vi "AMIMonitor.vi"() -> ()   [LabVIEW 2018]
uses:
  Global/Global Variables/Data_Display_global.vi
  Instrument_Setup.vi
panel:
  out "Numeric":i32
  out "Field set":bool
  out "Field rates set":bool=TRUE
  out "error out":errorcluster
  in  "error in (no error)":errorcluster
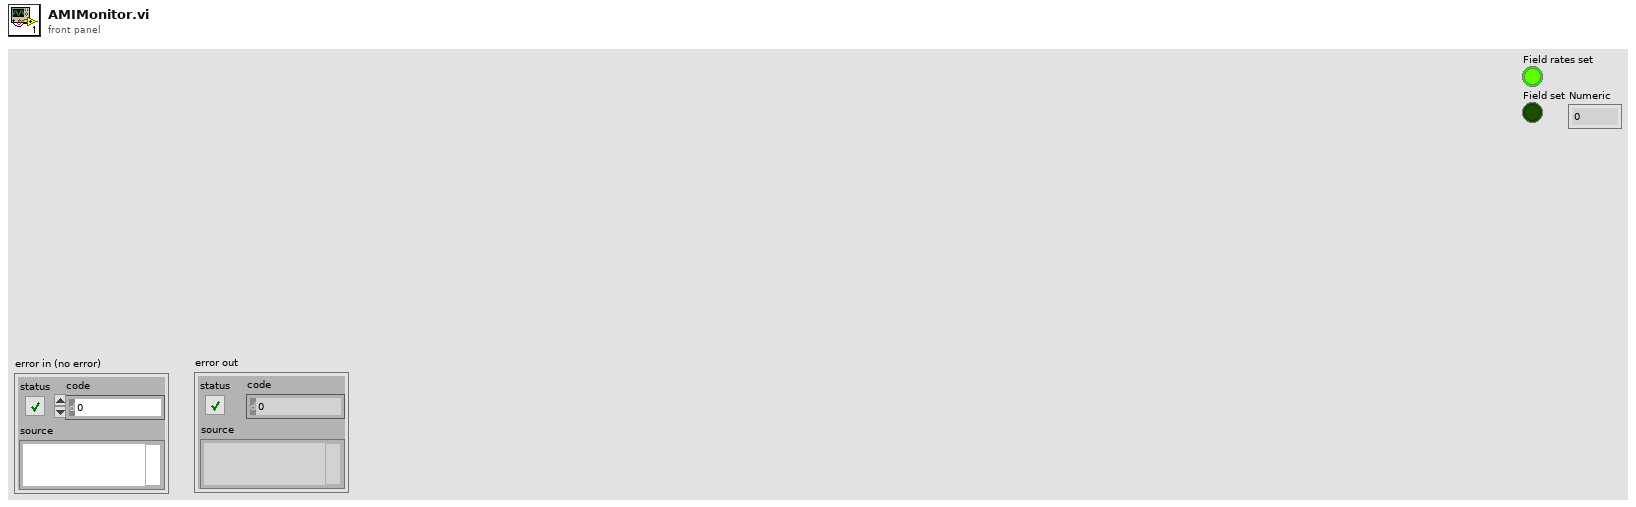
[diagram p1: front panel]
types:
  T1 = cluster{"GPIB address":i16, "GPIB bus":i16, "connection ID":refnum<k5>, "IP":string, "Active Comm Interface":u16, "Serial Port":refnum<visa-resource-name>, "Programmer Type":u16}
  T2 = cluster{"error":bool, "code":i32, "source":string}
  T3 = enum16{"", "RAMPING", "HOLDING", "PAUSED", "MANUAL UP", "MANUAL DOWN", "ZEROING CURRENT", "QUENCH DETECTED", "HEATING SWITCH", "AT ZER0", "COOLING SWITCH"}
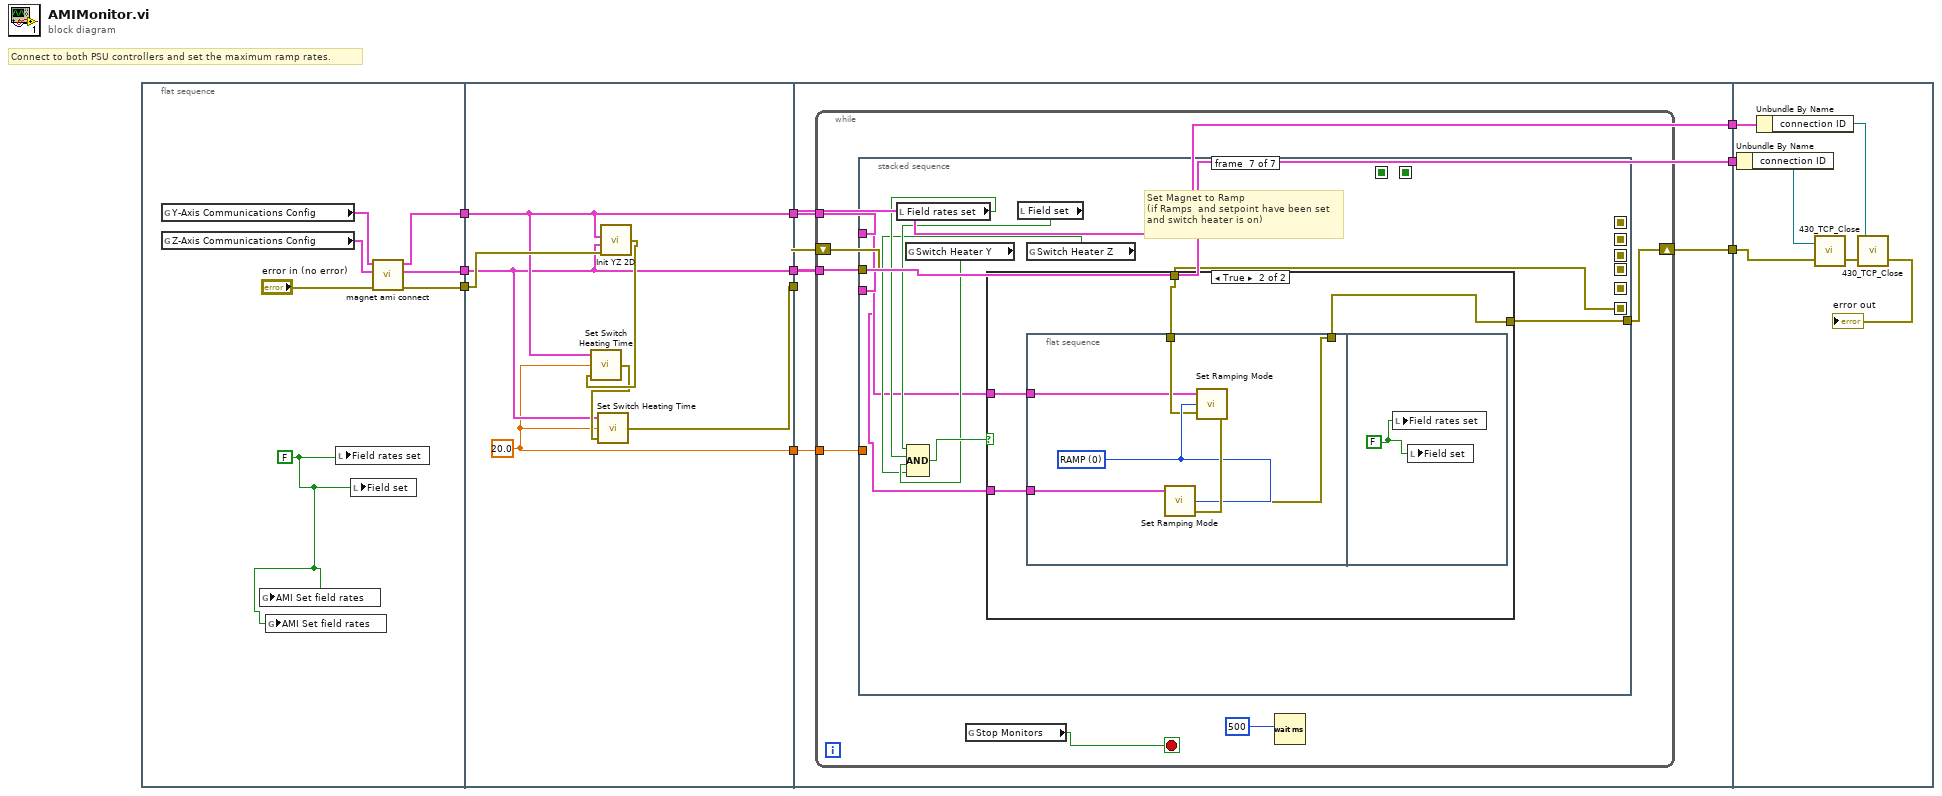
[diagram p0: block diagram]
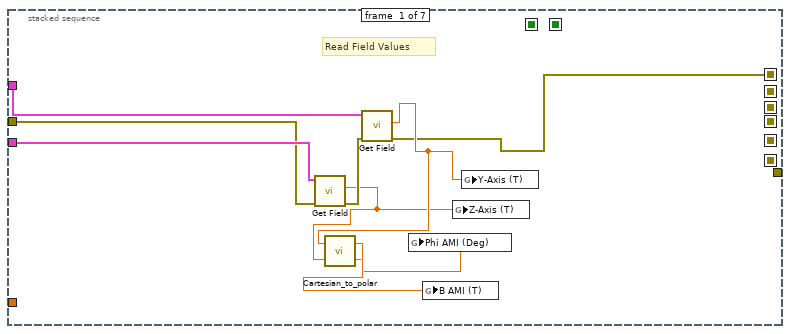
[diagram p2: hidden frame]
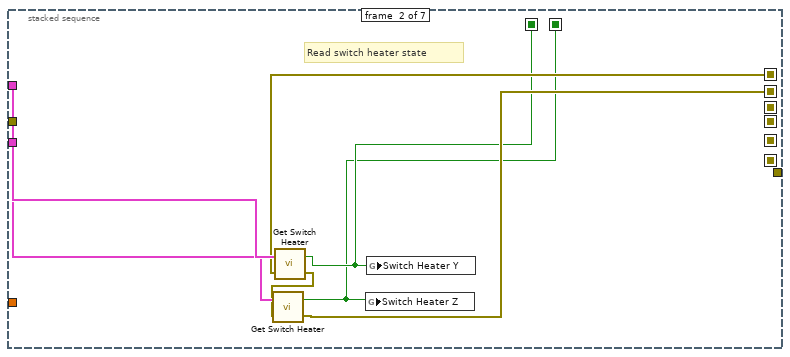
[diagram p3: hidden frame]
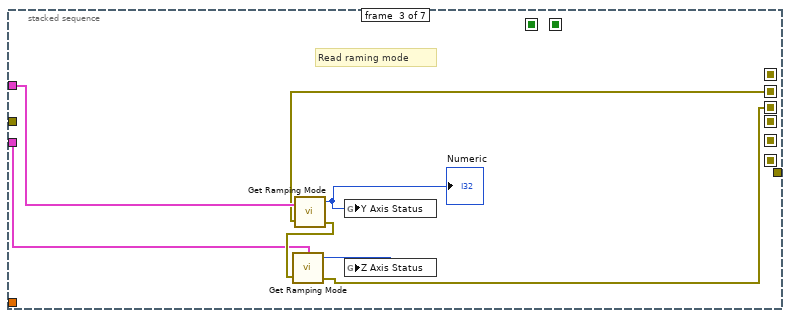
[diagram p4: hidden frame]
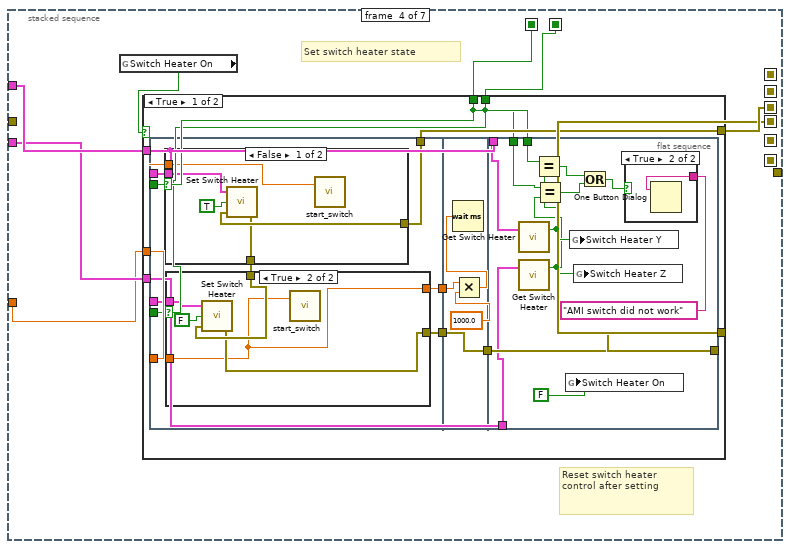
[diagram p5: hidden frame]
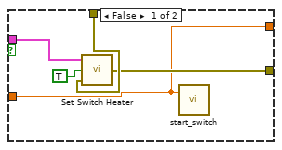
[diagram p6: hidden frame]
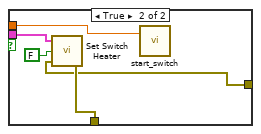
[diagram p7: hidden frame]
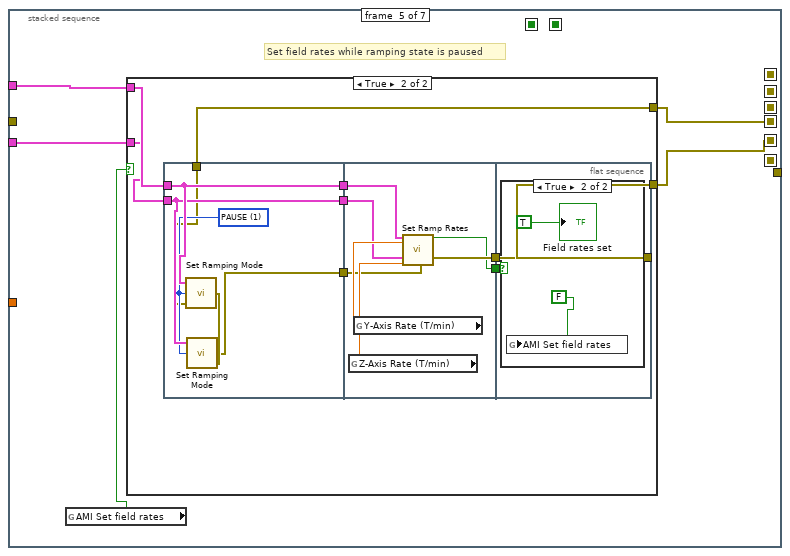
[diagram p10: hidden frame]
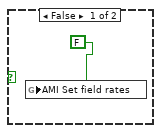
[diagram p12: hidden frame]
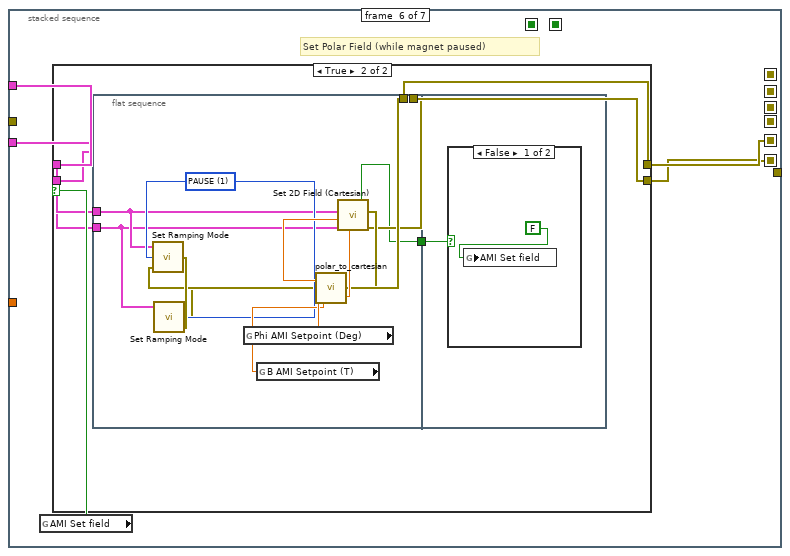
[diagram p13: hidden frame]
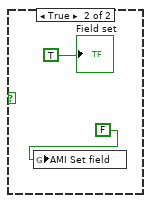
[diagram p15: hidden frame]
diagram:
  # "Connect to both PSU controllers and set the maximum ramp rates."
  n1 = flat-sequence {
    tunnel: [w14] -> w10
    tunnel: [w13] -> w8
    tunnel: [w12] -> w6
    tunnel: w10 -> [w23]
    tunnel: [w23] -> w9
    tunnel: w8 -> [w19]
    tunnel: [w19] -> w7
    tunnel: w6 -> [w24]
    tunnel: [w20] -> w5
    tunnel: [w18] -> w1
    tunnel: w9 -> [w28]
    tunnel: w7 -> [w27]
    tunnel: w5 -> [w29]
    tunnel: [w28] -> w4
    tunnel: [w27] -> w3
    tunnel: [w26] -> w2
    tunnel: w1 -> [w25]
    tunnel: w4 -> [w208]
    tunnel: w3 -> [w207]
    tunnel: w2 -> [w206]
    frame #0 {
      w11 = FALSE
      n2 = global read "Instrument_Setup.vi" "Y-Axis Communications Config"() -> (w17:T1)
      n3 = global read "Instrument_Setup.vi" "Z-Axis Communications Config"() -> (w16:T1)
      n4 = global write "Data_Display_global.vi" "AMI Set field rates"(w11) -> ()
      n5 = global write "Data_Display_global.vi" "AMI Set field rates"(w11) -> ()
      n6 = local write "Field rates set"(w11) -> ()
      n7 = local write "Field set"(w11) -> ()
      n8 = call "magnet ami connect.vi"("error in (no error)"="error in (no error)", "Z-Axis Communications Config"=w16, "Y-Axis Communications Config"=w17) -> ("error out"=w12:errorcluster, "Z-Axis Communications Config Out"=w13:T1, "Y-Axis Communications Config Out"=w14:T1)  [unwired: 6 in]
    }
    frame #1 {
      w18 = 20.0
      n9 = call "Init YZ 2D.vi"("error in"=w24, "Z-Axis Communications Config"=w19, "Y-Axis Communications Config"=w23) -> ("error out"=w22:T2)  [unwired: 7 in]
      n10 = call "Set Switch Heating Time.vi"("error in"=w22, "Switch Heating Time (sec)"=w18, "Communications Config"=w23) -> ("error out"=w21:T2)
      n11 = call "Set Switch Heating Time.vi"("error in"=w21, "Switch Heating Time (sec)"=w18, "Communications Config"=w19) -> ("error out"=w20:T2)
    }
    frame #2 {
      n12 = while {
        tunnel: w28 -> [w36]
        tunnel: w27 -> [w35]
        shift-right: [w30] -> w26
        shift-left: w29 -> [w34]
        tunnel: w25 -> [w31]
        stop <- w33 stop-if-true
        n13 = stacked-sequence {
          seq-local: [w37 _ _ _ _ _ _] -> [_ w50 _ _ _ _ _]
          seq-local: [_ _ _ w60 _ _ _] -> [_ _ _ _ w126 _ _]
          seq-local: [_ w48 _ _ _ _ _] -> [_ _ w55 _ _ _ _]
          seq-local: [_ w47 _ _ _ _ _] -> [_ _ _ w63 _ _ _]
          seq-local: [_ w46 _ _ _ _ _] -> [_ _ _ w62 _ _ _]
          seq-local: [_ _ w54 _ _ _ _] -> [_ _ _ w61 _ _ _]
          seq-local: [_ _ _ _ w125 _ _] -> [_ _ _ _ _ w159 _]
          seq-local: [_ _ _ _ _ w158 _] -> [_ _ _ _ _ _ w193]
          tunnel: w36 -> [w45 w52 w58 w66 w128 w162 w186]
          tunnel: w35 -> [w44 w51 w57 w65 w129 w161 w185]
          tunnel: w34 -> [w42 _ _ _ _ _ _]
          tunnel: w31 -> [_ _ _ w64 _ _ _]
          tunnel: [_ _ _ _ _ _ w192] -> w30
          frame #0 {
            # "Read Field Values"
            n14 = call "Get Field.vi"("Z-Axis Communications Config"=w44, "error in"=w42) -> ("Field(T)"=w40:dbl, "error out"=w43:T2)  [unwired: 4 in, 1 out]
            n15 = call "Get Field.vi"("Z-Axis Communications Config"=w45, "error in"=w43) -> ("Field(T)"=w41:dbl, "error out"=w37:T2)  [unwired: 4 in, 1 out]
            n16 = call "Cartesian_to_polar.vi"("Z-Axis (T)"=w40, "Y-Axis (T)"=w41) -> ("phi (deg)"=w38:dbl, "Radial (r) Field (T)"=w39:dbl)
            n17 = global write "Data_Display_global.vi" "Phi AMI (Deg)"(w38) -> ()
            n18 = global write "Data_Display_global.vi" "B AMI (T)"(w39) -> ()
            n19 = global write "Data_Display_global.vi" "Z-Axis (T)"(w40) -> ()
            n20 = global write "Data_Display_global.vi" "Y-Axis (T)"(w41) -> ()
          }
          frame #1 {
            # "Read switch heater state"
            n21 = call "Get Switch Heater.vi"("error in"=w50, "Communications Config"=w52) -> ("error out"=w49:T2, "Switch Heater Indicator"=w47:bool)
            n22 = call "Get Switch Heater.vi"("error in"=w49, "Communications Config"=w51) -> ("error out"=w48:T2, "Switch Heater Indicator"=w46:bool)
            n23 = global write "Data_Display_global.vi" "Switch Heater Z"(w46) -> ()
            n24 = global write "Data_Display_global.vi" "Switch Heater Y"(w47) -> ()
          }
          frame #2 {
            # "Read raming mode"
            n25 = call "Get Ramping Mode.vi"("Communications Config"=w58, "error in"=w55) -> ("Ramping Mode"=w53:T3, "error out"=w59:T2)  [unwired: 1 out]
            "Numeric" <- w53
            n26 = call "Get Ramping Mode.vi"("Communications Config"=w57, "error in"=w59) -> ("Ramping Mode"=w56:T3, "error out"=w54:T2)  [unwired: 1 out]
            n27 = global write "Data_Display_global.vi" "Y Axis Status"(w53) -> ()
            n28 = global write "Data_Display_global.vi" "Z Axis Status"(w56) -> ()
          }
          frame #3 {
            # "Reset switch heater \ncontrol after setting"
            # "Set switch heater state"
            n29 = global read "Data_Display_global.vi" "Switch Heater On"() -> (w67:bool)
            n30 = case shown="True" w67 {
              tunnel: w66 -> [w71 _]
              tunnel: w65 -> [w70 _]
              tunnel: w64 -> [w77 _]
              tunnel: w61 -> [w75 w124]
              tunnel: w63 -> [w69 _]
              tunnel: w62 -> [w68 _]
              tunnel: [w74 w124] -> w60
              frame True {
                n31 = flat-sequence {
                  tunnel: w71 -> [w86]
                  tunnel: w70 -> [w85]
                  tunnel: w77 -> [w82]
                  tunnel: [w83] -> w76
                  tunnel: w75 -> [w81]
                  tunnel: w69 -> [w80]
                  tunnel: w68 -> [w79]
                  tunnel: [w78] -> w73
                  tunnel: w76 -> [w110]
                  tunnel: w73 -> [w108]
                  tunnel: [w110] -> w72
                  tunnel: [w122] -> w74
                  tunnel: w72 -> [w122]
                  tunnel: w71 -> [w120]
                  tunnel: w70 -> [w119]
                  tunnel: w69 -> [w118]
                  tunnel: w68 -> [w117]
                  frame #0 {
                    n32 = case shown="False" w80 {
                      tunnel: w86 -> [w101 w105]
                      tunnel: w81 -> [w99 w102]
                      tunnel: [w98 w103] -> w84
                      tunnel: w82 -> [w97 w104]
                      frame False {
                        n33 = call "Set Switch Heater.vi"("error in"=w99, "Switch Heater Control"=TRUE, "Communications Config"=w101) -> ("error out"=w98:T2)
                        n34 = call "start_switch.vi"("Switch heater time"=w97) -> ()  [unwired: 2 in]
                      }
                      frame True {
                        n35 = call "Set Switch Heater.vi"("error in"=w102, "Switch Heater Control"=FALSE, "Communications Config"=w105) -> ("error out"=w103:T2)
                        n36 = call "start_switch.vi"("Switch heater time"=w104) -> ()  [unwired: 2 in]
                      }
                    }
                    n37 = case shown="True" w79 {
                      tunnel: w85 -> [w91 w93]
                      tunnel: w84 -> [w89 w95]
                      tunnel: [w88 w94] -> w83
                      tunnel: w82 -> [w87 w92]
                      tunnel: [w87 w92] -> w78
                      frame False {
                        n38 = call "Set Switch Heater.vi"("error in"=w89, "Switch Heater Control"=TRUE, "Communications Config"=w91) -> ("error out"=w88:T2)
                        n39 = call "start_switch.vi"("Switch heater time"=w87) -> ()  [unwired: 2 in]
                      }
                      frame True {
                        n40 = call "Set Switch Heater.vi"("error in"=w95, "Switch Heater Control"=FALSE, "Communications Config"=w93) -> ("error out"=w94:T2)
                        n41 = call "start_switch.vi"("Switch heater time"=w92) -> ()  [unwired: 2 in]
                      }
                    }
                  }
                  frame #1 {
                    n42 = Multiply(x=w108, y=1000.0) -> (x*y=w107:dbl)
                    n43 = Wait (ms)(milliseconds to wait=w107) -> ()  [unwired: 1 out]
                  }
                  frame #2 {
                    n44 = call "Get Switch Heater.vi"("Communications Config"=w120) -> ("Switch Heater Indicator"=w116:bool)  [unwired: 1 in, 1 out]
                    n45 = call "Get Switch Heater.vi"("Communications Config"=w119) -> ("Switch Heater Indicator"=w115:bool)  [unwired: 1 in, 1 out]
                    n46 = Equal?(x=w118, y=w116) -> (x = y?=w114:bool)
                    n47 = Equal?(x=w117, y=w115) -> (x = y?=w113:bool)
                    n48 = global write "Data_Display_global.vi" "Switch Heater On"(FALSE) -> ()
                    n49 = global write "Data_Display_global.vi" "Switch Heater Y"(w116) -> ()
                    n50 = global write "Data_Display_global.vi" "Switch Heater Z"(w115) -> ()
                    n51 = Or(x=w114, y=w113) -> (x .or. y?=w112:bool)
                    n52 = case shown="True" w112 {
                      tunnel: "AMI switch did not work" -> [_ w123]
                      frame False {
                      }
                      frame True {
                        n53 = One Button Dialog(message=w123) -> ()  [unwired: 1 in, 1 out]
                      }
                    }
                  }
                }
              }
              frame False {
              }
            }
          }
          frame #4 {
            # "Set field rates while ramping state is paused"
            n54 = global read "Data_Display_global.vi" "AMI Set field rates"() -> (w127:bool)
            n55 = case shown="True" w127 {
              tunnel: w129 -> [_ w135]
              tunnel: w128 -> [_ w137]
              tunnel: [w130 w139] -> w125
              tunnel: w126 -> [w130 w133]
              frame False {
              }
              frame True {
                n56 = flat-sequence {
                  tunnel: w137 -> [w144]
                  tunnel: [w144] -> w136
                  tunnel: w135 -> [w143]
                  tunnel: [w143] -> w134
                  tunnel: w133 -> [w141]
                  tunnel: [w140] -> w132
                  tunnel: [w150] -> w138
                  tunnel: w136 -> [w149]
                  tunnel: w134 -> [w148]
                  tunnel: w132 -> [w147]
                  tunnel: [w146] -> w131
                  tunnel: [w154] -> w139
                  tunnel: w138 -> [w154]
                  tunnel: w131 -> [w153]
                  frame #0 {
                    w142 = u16 1 items=["RAMP", "PAUSE", "Manual UP", "MANUAL DOWN", "ZERO"] ("Ramping Mode")
                    n57 = call "Set Ramping Mode.vi"("error in"=w141, "Ramping Mode"=w142, "Communications Config"=w144) -> ("error out"=w145:T2)
                    n58 = call "Set Ramping Mode.vi"("error in"=w145, "Ramping Mode"=w142, "Communications Config"=w143) -> ("error out"=w140:T2)
                  }
                  frame #1 {
                    n59 = global read "Data_Display_global.vi" "Z-Axis Rate (T/min)"() -> (w151:dbl)
                    n60 = global read "Data_Display_global.vi" "Y-Axis Rate (T/min)"() -> (w152:dbl)
                    n61 = call "Set Ramp Rates.vi"("Y-Axis Communications Config"=w149, "Y Rate (T/min)"=w152, "Z-Axis Communications Config"=w148, "Z Rate (T/min)"=w151, "error in"=w147) -> ("within limits?"=w146:bool, "error out"=w150:T2)  [unwired: 13 in]
                  }
                  frame #2 {
                    n62 = case shown="True" w153 {
                      frame False {
                        n63 = global write "Data_Display_global.vi" "AMI Set field rates"(FALSE) -> ()
                      }
                      frame True {
                        n64 = global write "Data_Display_global.vi" "AMI Set field rates"(FALSE) -> ()
                        "Field rates set" <- TRUE
                      }
                    }
                  }
                }
              }
            }
          }
          frame #5 {
            # "Set Polar Field (while magnet paused)"
            n65 = global read "Data_Display_global.vi" "AMI Set field"() -> (w160:bool)
            n66 = case shown="True" w160 {
              tunnel: w162 -> [_ w168]
              tunnel: w161 -> [_ w167]
              tunnel: [w163 w165] -> w158
              tunnel: w159 -> [w163 w166]
              frame False {
              }
              frame True {
                n67 = flat-sequence {
                  tunnel: w168 -> [w174]
                  tunnel: w167 -> [w173]
                  tunnel: w166 -> [w172]
                  tunnel: [w170] -> w165
                  tunnel: [w169] -> w164
                  tunnel: w164 -> [w181]
                  frame #0 {
                    w175 = u16 1 items=["RAMP", "PAUSE", "MANUAL UP", "MANUAL DOWN", "ZERO"] ("Ramping Mode")
                    n68 = call "Set Ramping Mode.vi"("error in"=w172, "Ramping Mode"=w175, "Communications Config"=w174) -> ("error out"=w176:T2)
                    n69 = call "Set Ramping Mode.vi"("error in"=w176, "Ramping Mode"=w175, "Communications Config"=w173) -> ("error out"=w171:T2)
                    n70 = global read "Data_Display_global.vi" "Phi AMI Setpoint (Deg)"() -> (w178:dbl)
                    n71 = global read "Data_Display_global.vi" "B AMI Setpoint (T)"() -> (w177:dbl)
                    n72 = call "polar_to_cartesian.vi"("B (T)"=w177, "Phi (Deg)"=w178) -> ("Z Field (T)"=w179:dbl, "Y Field (T)"=w180:dbl)
                    n73 = call "Set 2D Field (Cartesian).vi"("error in"=w171, "Z-Axis Field (T)"=w179, "Z-Axis Communications Config"=w173, "Y-Axis Field (T)"=w180, "Y-Axis Communications Config"=w174) -> ("error out"=w170:T2, "Within Limits?"=w169:bool)  [unwired: 3 in]
                  }
                  frame #1 {
                    n74 = case shown="False" w181 {
                      frame False {
                        n75 = global write "Data_Display_global.vi" "AMI Set field"(FALSE) -> ()
                      }
                      frame True {
                        n76 = global write "Data_Display_global.vi" "AMI Set field"(FALSE) -> ()
                        "Field set" <- TRUE
                      }
                    }
                  }
                }
              }
            }
          }
          frame #6 {
            # "Set Magnet to Ramp\n(if Ramps  and setpoint have been set\nand switch heater is on)"
            n77 = local read "Field rates set"() -> (w189:bool)
            n78 = global read "Data_Display_global.vi" "Switch Heater Y"() -> (w188:bool)
            n79 = local read "Field set"() -> (w190:bool)
            n80 = global read "Data_Display_global.vi" "Switch Heater Z"() -> (w187:bool)
            n81 = Compound Arithmetic op=AND(w190, w189, w188, w187) -> (w191:bool)
            n82 = case shown="True" w191 {
              tunnel: w193 -> [w194 w198]
              tunnel: [w194 w197] -> w192
              tunnel: w186 -> [_ w196]
              tunnel: w185 -> [_ w195]
              frame False {
              }
              frame True {
                n83 = flat-sequence {
                  tunnel: w198 -> [w202]
                  tunnel: [w201] -> w197
                  tunnel: w196 -> [w200]
                  tunnel: w195 -> [w199]
                  frame #0 {
                    w203 = u16 0 items=["RAMP", "PAUSE", "MANUAL UP", "MANUAL DOWN", "ZERO"] ("Ramping Mode")
                    n84 = call "Set Ramping Mode.vi"("error in"=w202, "Ramping Mode"=w203, "Communications Config"=w200) -> ("error out"=w204:T2)
                    n85 = call "Set Ramping Mode.vi"("error in"=w204, "Ramping Mode"=w203, "Communications Config"=w199) -> ("error out"=w201:T2)
                  }
                  frame #1 {
                    w205 = FALSE
                    n86 = local write "Field rates set"(w205) -> ()
                    n87 = local write "Field set"(w205) -> ()
                  }
                }
              }
            }
          }
        }
        n88 = global read "Data_Display_global.vi" "Stop Monitors"() -> (w33:bool)
        n89 = Wait (ms)(milliseconds to wait=500) -> ()  [unwired: 1 out]
      }
    }
    frame #3 {
      n90 = Unbundle By Name(w207) -> ("connection ID"=w210:refnum<k5>)
      n91 = Unbundle By Name(w208) -> ("connection ID"=w209:refnum<k5>)
      n92 = call "430_TCP_Close.vi"("error in (no error)"=w206, "connection ID"=w210) -> ("error out"=w211:errorcluster)  [unwired: 1 out]
      n93 = call "430_TCP_Close.vi"("error in (no error)"=w211, "connection ID"=w209) -> ("error out"=→"error out":errorcluster)  [unwired: 1 out]
    }
  }
